vi "CreateCSVWithFirstRshTest.vi"() -> ()   [LabVIEW 2017]
uses:
  <vilib>/Utility/file.llb/Read Delimited Spreadsheet (DBL).vi
panel:
  in  "element":dbl
  in  "file path Rsh":path=path "C:/Users/Jonathan/Documents/UHasselt/Masterproef/LabVEIW/data/24-05-19_11h55/Module1/0.csv"
  out "error out 2":errorcluster
  in  "base path":path
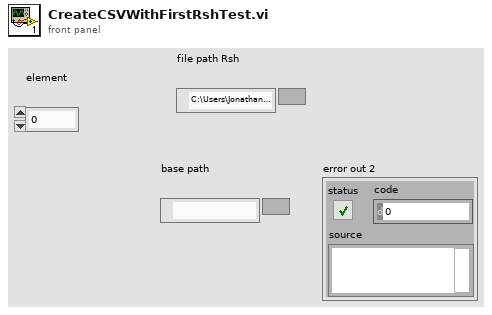
[diagram p1: front panel]
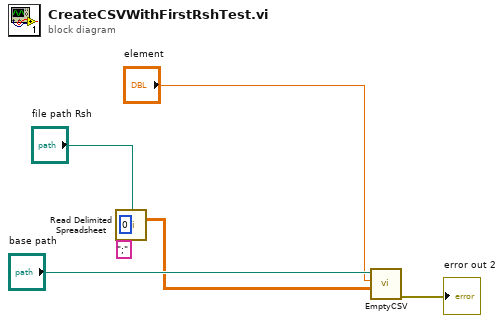
[diagram p0: block diagram]
diagram:
  n1 = call-poly <vilib>:"Read Delimited Spreadsheet.vi"("file path (dialog if empty)"="file path Rsh", "start of read offset (chars.:0)"=0, "delimiter (\\t)"=";" ("delimiter (\\t)")) -> ("all rows"=w2:dbl[][])  [unwired: 7 in, 5 out]
  n2 = call "EmptyCSV.vi"("all rows"=w2, "element"="element", "base path"="base path") -> ("error out"=→"error out 2":errorcluster)  [unwired: 8 in]
